vi "Knob Fill (One-Way).vi"(9 "Value":dbl, 10 "Maximum":dbl, 11 "Minimum":dbl) -> (3 "Marker Values":cluster{"Value":dbl, "Color Box":u32}[](array[cluster]))   [LabVIEW 2019, in "User Interface.lvlib"]
doc: "Logic for a one-way marker fill, from min to max."
uses:
  User Interface.lvlib
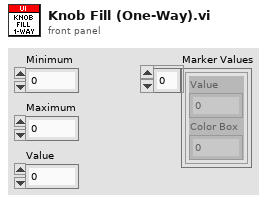
[diagram p1: front panel]
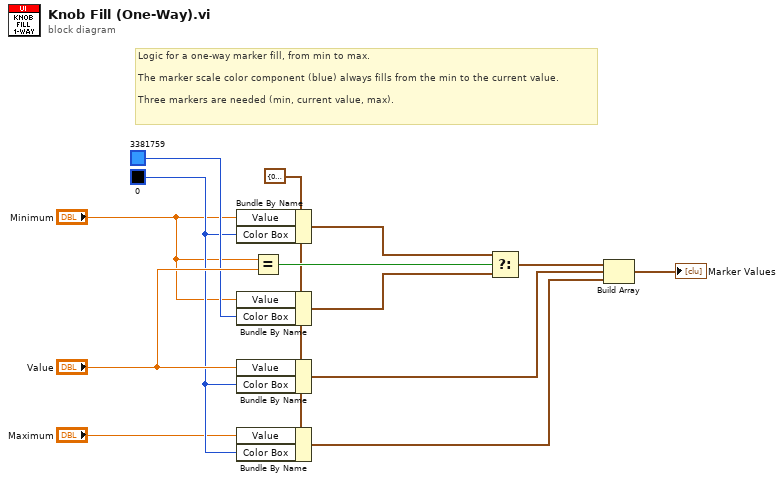
[diagram p0: block diagram]
diagram:
  w4 = cluster{"Value":dbl, "Color Box":u32} {"Value"=0.0, "Color Box"=0}
  w7 = u32 0 ("Color Box")
  # "Logic for a one-way marker fill, from min to max.\n\nThe marker scale color component (blue) always fills from the min to the current value.\n\nThree markers are needed (min, current value, max)."
  n1 = Bundle By Name(cluster=w4, "Value"="Minimum", "Color Box"=w7) -> (w11:cluster{"Value":dbl, "Color Box":u32})
  n2 = Bundle By Name(cluster=w4, "Value"="Minimum", "Color Box"=u32 3381759) -> (w10:cluster{"Value":dbl, "Color Box":u32})
  n3 = Bundle By Name(cluster=w4, "Value"="Value", "Color Box"=w7) -> (w6:cluster{"Value":dbl, "Color Box":u32})
  n4 = Bundle By Name(cluster=w4, "Value"="Maximum", "Color Box"=w7) -> (w5:cluster{"Value":dbl, "Color Box":u32})
  n5 = Equal?(x="Minimum", y="Value") -> (x = y?=w13:bool)
  n6 = Select(t=w11, s=w13, f=w10) -> (s? t:f=w12:cluster{"Value":dbl, "Color Box":u32})
  n7 = Build Array(w12, w6, w5) -> (→"Marker Values":cluster{"Value":dbl, "Color Box":u32}[])
